vi "Byte Buffer.Mapping.Get Required Buffer Size.vi"(11 "mappings":T1[](array[typedef])) -> (2 "required buffer size":i32, 3 "mappings dup":T1[](array[typedef]))   [LabVIEW 2016, in "VeriStand Data.lvlib" / "Byte Buffer.lvclass"]
uses:
  Byte Buffer.lvclass
  Byte Buffer.Mapping.ctl
  Typedefs/Typedefs.Data Types.ctl
  SubVIs/Sizeof.Scalar.vi
  VeriStand Data.lvlib
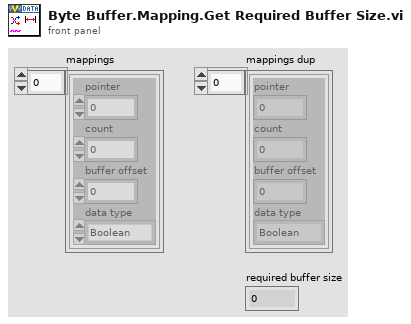
[diagram p1: front panel]
types:
  T1 = typedef "VeriStand Data.lvlib/Byte Buffer.lvclass/Byte Buffer.Mapping.ctl" = cluster{"pointer":u64, "count":i32, "buffer offset":i32, "data type":T2}
  T2 = typedef "VeriStand Data.lvlib/Typedefs.Data Types.ctl" = enum16{"Boolean", "Single", "Double", "I8", "I16", "I32", "I64", "U8", "U16", "U32", "U64"}
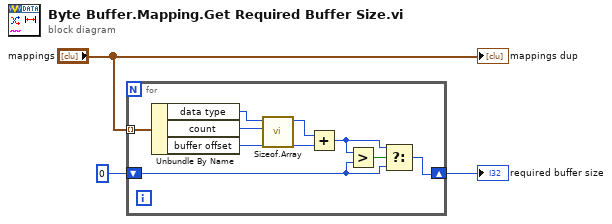
[diagram p0: block diagram]
diagram:
  n1 = for {
    tunnel: "mappings" -> [w12] mode=indexing
    shift-right: [w4] -> w1
    shift-left: 0 ("x+y") -> [w5]
    n2 = Unbundle By Name(w12) -> ("data type"=w8:T2, "count"=w7:i32, "buffer offset"=w6:i32)
    n3 = call "Sizeof.Array.vi"("count"=w7, "data type"=w8) -> ("size"=w10:i32)  [unwired: 9 in]
    n4 = Add(x=w10, y=w6) -> (x+y=w9:i32)
    n5 = Greater?(x=w9, y=w5) -> (0:w11:bool)
    n6 = Select(t=w9, s=w11, f=w5) -> (s? t:f=w4:i32)
  }
  "required buffer size" <- w1
  "mappings dup" <- "mappings"
